vi "set Active VIs.vi"(8 "error in (no error)":errorcluster, 10 "Active VI":refnum<vi>[](array[refnum]), 11 "VI Collection in":refnum<class "VI Collection.lvclass">) -> (0 "error out":errorcluster, 3 "VI Collection out":refnum<class "VI Collection.lvclass">)   [LabVIEW 2015, in "QuickVIew.lvlib" / "VI Collection.lvclass"]
doc: "TLB Prime - Application Template 1.3.0.24\nNorm Kirchner, NI Systems Engineering - NI\nCopyright (c) 2014, NI"
uses:
  VI Collection.lvclass
  VI Collection.lvclass/VI Collection.ctl
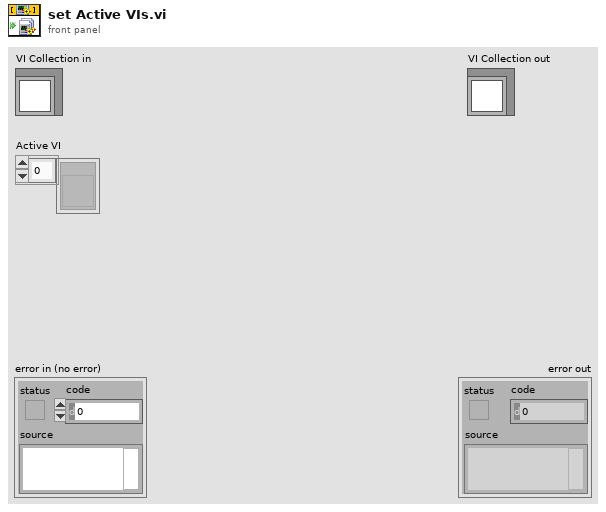
[diagram p1: front panel]
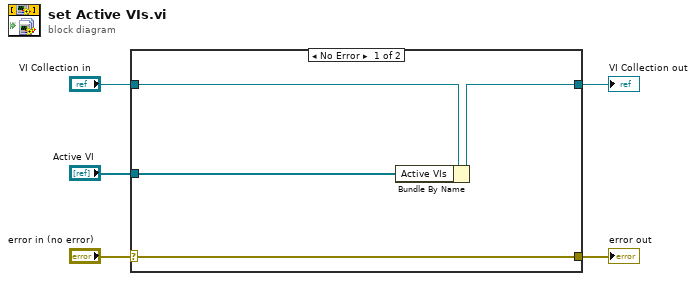
[diagram p0: block diagram]
diagram:
  n1 = case shown="No Error" "error in (no error)" {
    selector: "error in (no error)" -> [w9 w10]
    tunnel: [w9 w10] -> w4
    tunnel: [w6 w11] -> w2
    tunnel: "VI Collection in" -> [w8 w11]
    tunnel: "Active VI" -> [w7 _]
    frame No Error {
      n2 = Bundle By Name(cluster=w8, "Active VIs"=w7) -> (w6:refnum<class "VI Collection.lvclass">)
    }
    frame Error {
    }
  }
  "error out" <- w4
  "VI Collection out" <- w2
